vi "Initialize.vi"(1 "FPS":u32=30, 2 "Path":path, 3 "Size":T2, 4 "Type":T1=16 items=["Grayscale U8"=0, "Grayscale U16"=2, "Grayscale Single"=5, "Grayscale Double"=6, "RGB U8"=16], 5 "error in (no error)":errorcluster, 9 "FourCC Codec":string="0") -> (14 "video writer out":refnum<class "MSC Video Writer.lvclass">, 19 "error out":errorcluster)   [LabVIEW 2014, in "MSC Video Writer.lvclass"]
doc: "Initializes a Video Writer Object to save a video on the HD.\nUse the FourCC Codec to specify video compression settings. \"0\" stands for uncompressed and \"-1\" opens a dialogue."
uses:
  MSC Video Writer.lvclass
  MSC Image_class/controls/Size.ctl
  MSC Image_class/controls/Image Type.ctl
  controls/Video Writer.ctl
  MSC Video Writer.lvclass/MSC Video Writer.ctl
  MSC Image_class/MSC Image.lvclass
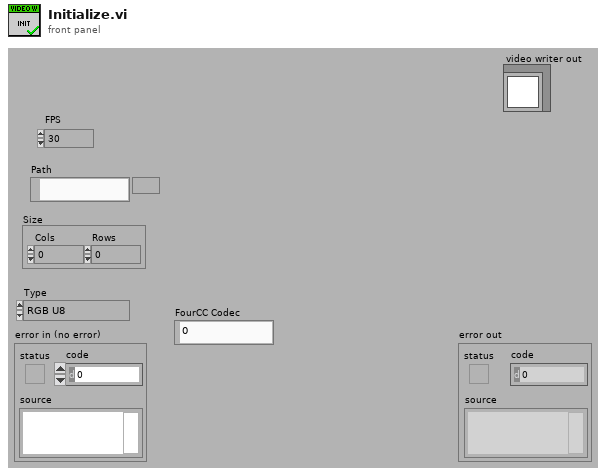
[diagram p1: front panel]
types:
  T1 = typedef "MSC Image.lvclass/Image Type.ctl" = i32
  T2 = typedef "MSC Image.lvclass/Size.ctl" = cluster{"Cols":i32, "Rows":i32}
  T3 = typedef "MSC Video Writer.lvclass/Video Writer.ctl" = cluster{"Pointer":u64, "FPS":u32, "Path":path, "FourCC Codec":string, "Size":T2, "Type":T1}
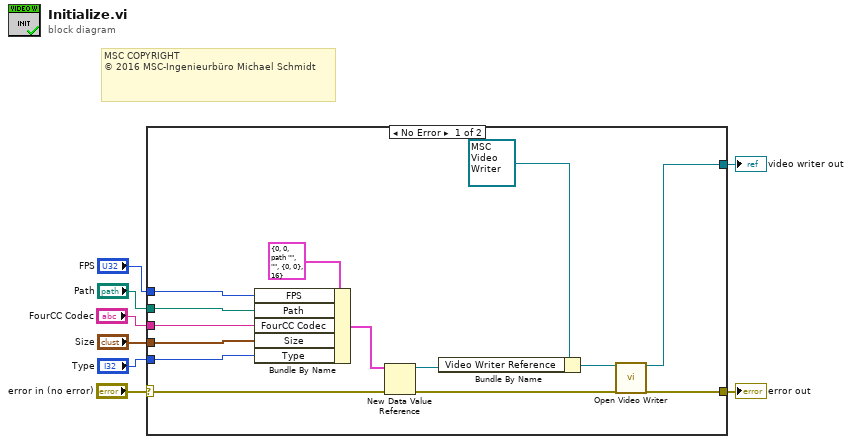
[diagram p0: block diagram]
diagram:
  # "MSC COPYRIGHT\n© 2016 MSC-Ingenieurbüro Michael Schmidt"
  # "MSC COPYRIGHT\n© 2016 MSC-Ingenieurbüro Michael Schmidt"
  n1 = case shown="No Error" "error in (no error)" {
    selector: "error in (no error)" -> [w21 w23]
    tunnel: [w14 _] -> w8
    tunnel: [w12 w23] -> w6
    tunnel: "FPS" -> [w19 _]
    tunnel: "Path" -> [w18 _]
    tunnel: "FourCC Codec" -> [w10 _]
    tunnel: "Size" -> [w16 _]
    tunnel: "Type" -> [w11 _]
    frame No Error {
      n2 = Bundle By Name(cluster=T3 {"Pointer"=0, "FPS"=0, "Path"=path "", "FourCC Codec"="", "Size"={"Cols"=0, "Rows"=0}, "Type"=16} ("Video Writer"), "FPS"=w19, "Path"=w18, "FourCC Codec"=w10, "Size"=w16, "Type"=w11) -> (w22:T3)
      n3 = New Data Value Reference(data value=w22, error in=w21) -> (data value reference=w17:refnum<data-value>, error out=w13:errorcluster)
      n4 = Bundle By Name(cluster=refnum<class "MSC Video Writer.lvclass"> refnum ("video writer out"), "Video Writer Reference"=w17) -> (w15:refnum<class "MSC Video Writer.lvclass">)
      n5 = call "Open Video Writer.vi"("video writer in"=w15, "error in (no error)"=w13) -> ("video writer out"=w14:refnum<class "MSC Video Writer.lvclass">, "error out"=w12:errorcluster)  [unwired: 16 in]
    }
    frame Error {
    }
  }
  "video writer out" <- w8
  "error out" <- w6
